vi "Acquisition Daemon.vi"(10 "Buffer size":i64, 11 "HRF_Device":refnum<class "HRF_Device.lvclass">) -> ()   [LabVIEW 2020, in "HRF_Device.lvclass"]
uses:
  HRF_Device.lvclass
  HRF_Device.lvclass/HRF_Device.ctl
  D:/work/HackRF/Labview Driver/NetHackrf.dll
  NetHackrf.dll
panel:
  out "error out":errorcluster
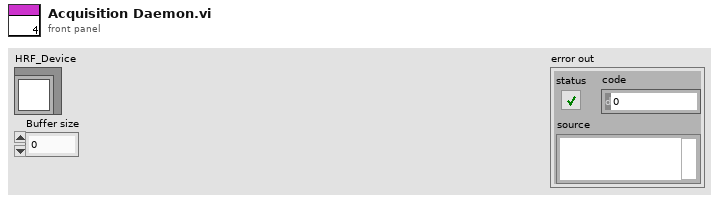
[diagram p1: front panel]
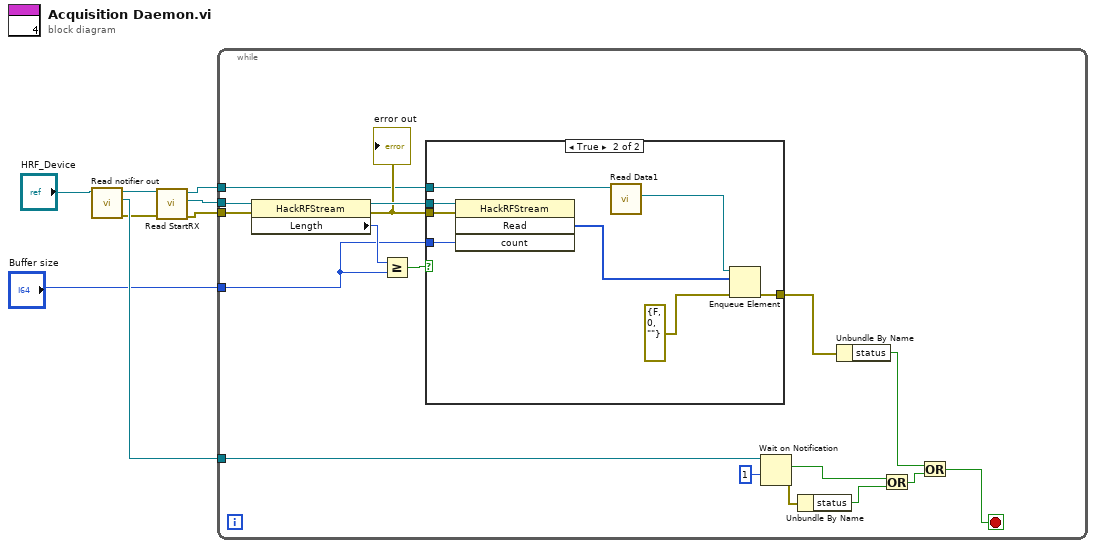
[diagram p0: block diagram]
diagram:
  n1 = call "Read notifier out.vi"("HRF_Device in"="HRF_Device") -> ("error out"=w2:errorcluster, "notifier out"=w4:refnum<notifier>, "HRF_Device out"=w5:refnum<class "HRF_Device.lvclass">)  [unwired: 8 in]
  n2 = call "Read StartRX.vi"("error in (no error)"=w2, "HRF_Device in"=w5) -> ("error out"=w1:errorcluster, "StartRX"=w8:refnum<k24>, "HRF_Device out"=w7:refnum<class "HRF_Device.lvclass">)  [unwired: 7 in]
  n3 = while {
    tunnel: w8 -> [w25]
    tunnel: w7 -> [w13]
    tunnel: w4 -> [w22]
    tunnel: "Buffer size" -> [w10]
    tunnel: w1 -> [w9]
    stop <- w15 stop-if-true
    n4 = property class="HackRFStream"(reference=w25, error in=w9) -> (reference out=w24:refnum<k24>, error out=w23:errorcluster, "Length"=w12:i64)
    "error out" <- w23
    n5 = Greater Or Equal?(x=w12, y=w10) -> (x >= y?=w11:bool)
    n6 = case shown="True" w11 {
      tunnel: w24 -> [_ w33]
      tunnel: w23 -> [_ w32]
      tunnel: [_ w30] -> w17
      tunnel: w13 -> [_ w28]
      tunnel: w10 -> [_ w26]
      frame False {
      }
      frame True {
        n7 = invoke class="HackRFStream" method="Read"(reference=w33, error in=w32, "count"=w26) -> ("Read"=w31:u8[])  [unwired: 1 in, 3 out]
        n8 = call "Read Data1.vi"("HRF_Device in"=w28) -> ("Data"=w27:refnum<queue>)  [unwired: 8 in, 2 out]
        n9 = Enqueue Element(queue=w27, element=w31, error in (no error)=errorcluster {"status"=FALSE, "code"=0, "source"=""} ("error out")) -> (error out=w30:errorcluster)  [unwired: 1 in, 2 out]
      }
    }
    n10 = Wait on Notification(notifier=w22, timeout in ms (-1)=1) -> (notification=w14:bool, error out=w20:errorcluster)  [unwired: 2 in, 2 out]
    n11 = Unbundle By Name(w20) -> ("status"=w19:bool)
    n12 = Unbundle By Name(w17) -> ("status"=w16:bool)
    n13 = Or(x=w14, y=w19) -> (x .or. y?=w18:bool)
    n14 = Or(x=w16, y=w18) -> (x .or. y?=w15:bool)
  }
